vi "Actor Core.vi"(8 "error in":errorcluster, 11 "Waveform Generator in":refnum<class "Waveform Generator.lvclass">) -> (0 "error out":errorcluster, 3 "Actor out":refnum<class "Actor.lvclass">)   [LabVIEW 2021, in "Waveform Generator.lvclass"]
doc: "(<B>Filename</B>: Actor Framework.lvlib:Actor.lvclass:Actor Core.vi)\n\nReceives messages to the actor, reacts to them, and initiates any error handling that may shut the actor down.\n\nDescendant classes may override this VI to append parallel tasks for the actor to complete while it handles messages. Overrides use the Call Parent Method node."
uses:
  Waveform Generator.lvclass
  <vilib>/ActorFramework/Actor/Actor.lvclass
  NHMFL_Core/Libraries/NI-DAQ/DAQmx Synthesizer/DAQmx Synthesizer Configuration.ctl
  Pulse Recorders/Pulse Recorder Actor/Pulse Recorder Actor.lvclass
  Waveform Generator.lvclass/Waveform Generator.ctl
panel:
  in  "Configuration":T1={"Channel names"=["Vout"], "Waveform file"=path "", "Ranges"=[10.0], "Post-trigger delay"=0.01, "Post-trigger duration"=0.1, "Rate"=1000000.0, "Re-name channels"=[], "Active channels"="0:1", "External\nclock"=FALSE, "Group name"="p"} {"Rate" format="%#_8pHz"; "Post-trigger duration" format="%#_6ps"; "Post-trigger delay" format="%#_6ps"; "Ranges" format="%#_6pV"}
  out "Done":bool
  out "Armed":bool
  out "Name":string
  # "Pulse config"
  # "Waveform generation config"
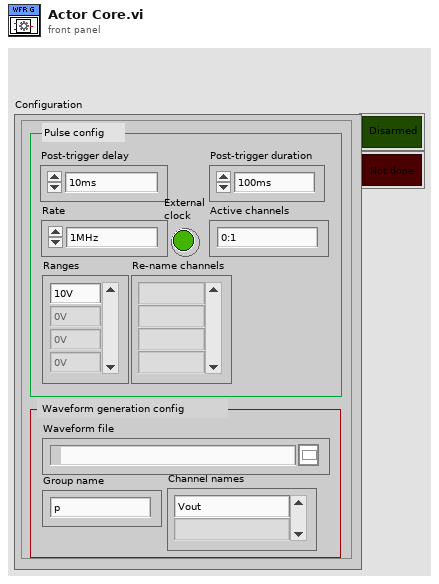
[diagram p1: front panel]
types:
  T1 = typedef "DAQmx Synthesizer Configuration.ctl" = cluster{"Channel names":string[], "Waveform file":path, "Ranges":dbl[], "Post-trigger delay":dbl, "Post-trigger duration":dbl, "Rate":dbl, "Re-name channels":string[], "Active channels":string, "External\nclock":bool, "Group name":string}
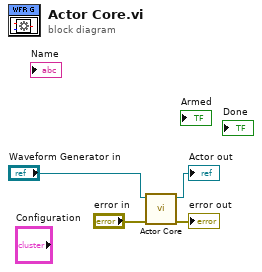
[diagram p0: block diagram]
diagram:
  n1 = call-parent "Actor Core.vi"("error in"="error in", "Pulse Recorder in"="Waveform Generator in") -> ("error out"=→"error out":errorcluster, "Actor out"=→"Actor out":refnum<class "Actor.lvclass">)  [unwired: 8 in]
